vi "readFromXML.vi"(8 "error in (no error)":errorcluster, 10 "XMLin":string=" <GuideMeasuredError>\n\t<tcsGuideCorrectionTime>15</tcsGuideCorrectionTime>\t\n\t<xError_mm>77</xError_mm>\n\t<trackID>1414.22</trackID>\n\t<yError_mm>88</yError_mm>\n  </GuideMeasuredError>", 11 "GuiderMeasuredError in":refnum<class "GuiderMeasuredError.lvclass">) -> (0 "error out":errorcluster, 3 "GuiderMeasuredError out":refnum<class "GuiderMeasuredError.lvclass">)   [LabVIEW 2022 SP3, in "TCSDataDefinitions.lvlib" / "TCSGuiderCommand.lvlib" / "GuiderMeasuredError.lvclass"]
uses:
  GuiderMeasuredError.lvclass
  <userlib>/Common/UnitsAndXML/FlattenItemWithUnitToXML/FlattenLengthToXML/LengthUnit.ctl
  GuiderMeasuredError.lvclass/GuiderMeasuredError.ctl
  TCSGuiderCommand/TCSGuiderCommand.lvclass
  <userlib>/Common/UnitsAndXML/UnitsAndXML.lvlib
  <userlib>/Common/XML/XMLParser/XMLParser.lvclass
panel:
  out "data":timestamp
  out "trackID":dbl=1414.22
  out "yError_mm":dbl[unit]=0.088
  out "xError_mm":dbl[unit]=0.077
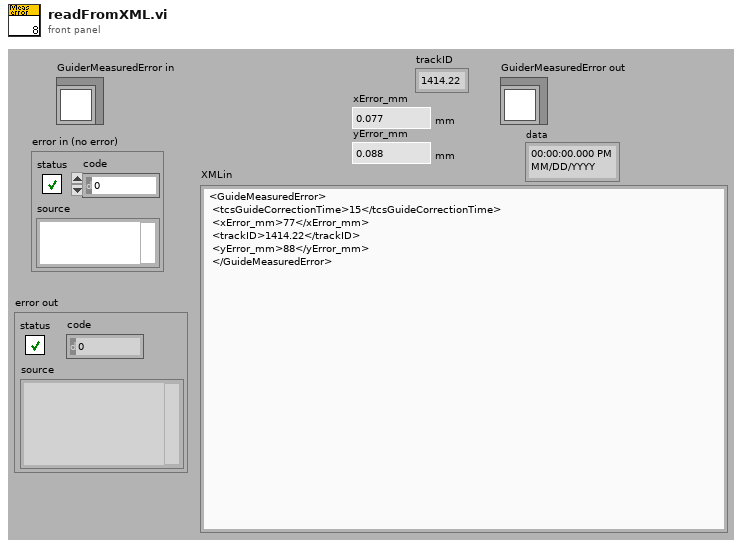
[diagram p1: front panel]
types:
  T1 = typedef "UnitsAndXML.lvlib/LengthUnit.ctl" = enum16{"m", "Angstrom", "AU", "chain", "cm", "cubit", "fathom", "fermi", "ft", "furlong", "hubble", "in", "ly", "mi", "mm", "rod", "um", "yd"}
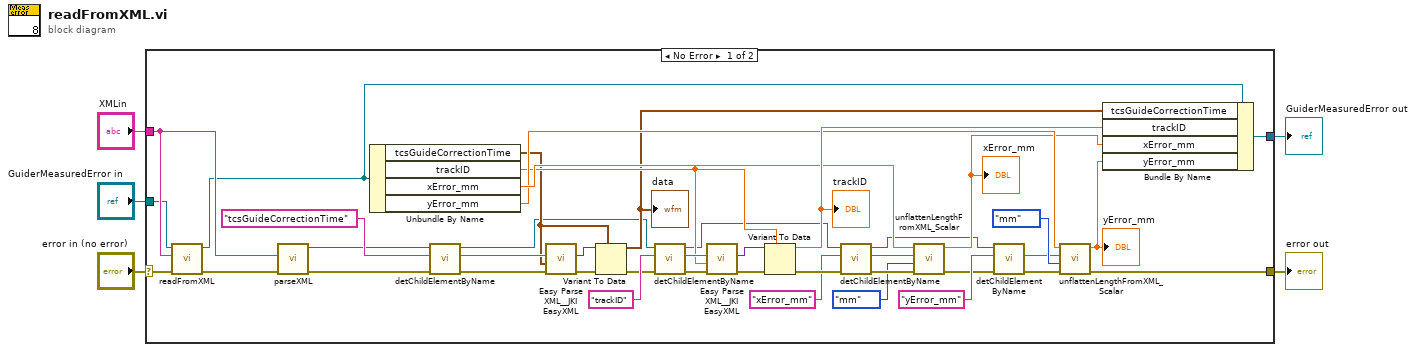
[diagram p0: block diagram]
diagram:
  n1 = case shown="No Error" "error in (no error)" {
    selector: "error in (no error)" -> [w42 w48]
    tunnel: [w23 w48] -> w4
    tunnel: [w43 w47] -> w2
    tunnel: "GuiderMeasuredError in" -> [w11 w47]
    tunnel: "XMLin" -> [w45 _]
    frame No Error {
      n2 = call-parent "readFromXML.vi"("error in (no error)"=w42, "XML in"=w45, "TCSGuiderCommand.lvclass"=w11) -> ("error out"=w44:errorcluster, "TCSGuiderCommand.lvclass 2"=w10:refnum<class "GuiderMeasuredError.lvclass">)  [unwired: 7 in]
      n3 = call <userlib>:"parseXML.vi"("error in (no error)"=w44, "XMLString in"=w45) -> ("error out"=w46:errorcluster, "Element out"=w9:refnum<class "XMLParser.lvclass">)  [unwired: 8 in]
      n4 = Unbundle By Name(w10) -> ("tcsGuideCorrectionTime"=w16:timestamp, "trackID"=w19:dbl, "xError_mm"=w30:dbl[unit], "yError_mm"=w22:dbl[unit])
      n5 = call <userlib>:"detChildElementByName.vi"("error in (no error)"=w46, "childName"="tcsGuideCorrectionTime" ("ChildName"), "Element in"=w9) -> ("error out"=w12:errorcluster, "childXML"=w18:string, "Element out"=w8:refnum<class "XMLParser.lvclass">)  [unwired: 5 in, 1 out]
      n6 = call <vilib>:"Easy Parse XML__JKI EasyXML.vi"("error in (no error)"=w12, "LabVIEW Data (Type)"=w16, "XML String"=w18) -> ("error out"=w14:errorcluster, "LabVIEW Data"=w17:variant)  [unwired: 7 in]
      n7 = Variant To Data(error in=w14, type=w16, Variant=w17) -> (data=w15:timestamp, error out=w13:errorcluster)
      "data" <- w15
      n8 = call <userlib>:"detChildElementByName.vi"("error in (no error)"=w13, "childName"="trackID" ("ChildName"), "Element in"=w8) -> ("error out"=w38:errorcluster, "childXML"=w39:string, "Element out"=w7:refnum<class "XMLParser.lvclass">)  [unwired: 5 in, 1 out]
      n9 = call <vilib>:"Easy Parse XML__JKI EasyXML.vi"("error in (no error)"=w38, "LabVIEW Data (Type)"=w19, "XML String"=w39) -> ("error out"=w36:errorcluster, "LabVIEW Data"=w37:variant)  [unwired: 7 in]
      n10 = Variant To Data(error in=w36, type=w19, Variant=w37) -> (data=w34:dbl, error out=w35:errorcluster)
      "trackID" <- w34
      n11 = call <userlib>:"detChildElementByName.vi"("error in (no error)"=w35, "childName"="xError_mm" ("ChildName"), "Element in"=w7) -> ("error out"=w29:errorcluster, "childXML"=w31:string, "Element out"=w6:refnum<class "XMLParser.lvclass">)  [unwired: 5 in, 1 out]
      n12 = call <userlib>:"unflattenLengthFromXML_Scalar.vi"("error in (no error)"=w29, "lengthUnitInXML"=LengthUnit."mm", "xmlString"=w31, "lengthForType"=w30) -> ("error out"=w25:errorcluster, "length"=w21:dbl[unit])  [unwired: 6 in]
      "xError_mm" <- w21
      n13 = call <userlib>:"detChildElementByName.vi"("error in (no error)"=w25, "childName"="yError_mm" ("ChildName"), "Element in"=w6) -> ("error out"=w24:errorcluster, "childXML"=w26:string)  [unwired: 5 in, 2 out]
      n14 = call <userlib>:"unflattenLengthFromXML_Scalar.vi"("error in (no error)"=w24, "lengthUnitInXML"=LengthUnit."mm", "xmlString"=w26, "lengthForType"=w22) -> ("error out"=w23:errorcluster, "length"=w20:dbl[unit])  [unwired: 6 in]
      "yError_mm" <- w20
      n15 = Bundle By Name(cluster=w10, "tcsGuideCorrectionTime"=w15, "trackID"=w34, "xError_mm"=w21, "yError_mm"=w20) -> (w43:refnum<class "GuiderMeasuredError.lvclass">)
    }
    frame Error {
    }
  }
  "error out" <- w4
  "GuiderMeasuredError out" <- w2
